vi "Main VI.vi"   [LabVIEW 2017]
uses:
  Main Flow.ctl
types:
  T1 = typedef "Main Flow.ctl" = enum16{"Initialize", "Calibrate Max Threshold", "Wait for Signal", "Convert Signal", "Noise Processing", "Threshold Processing", "Stop"}
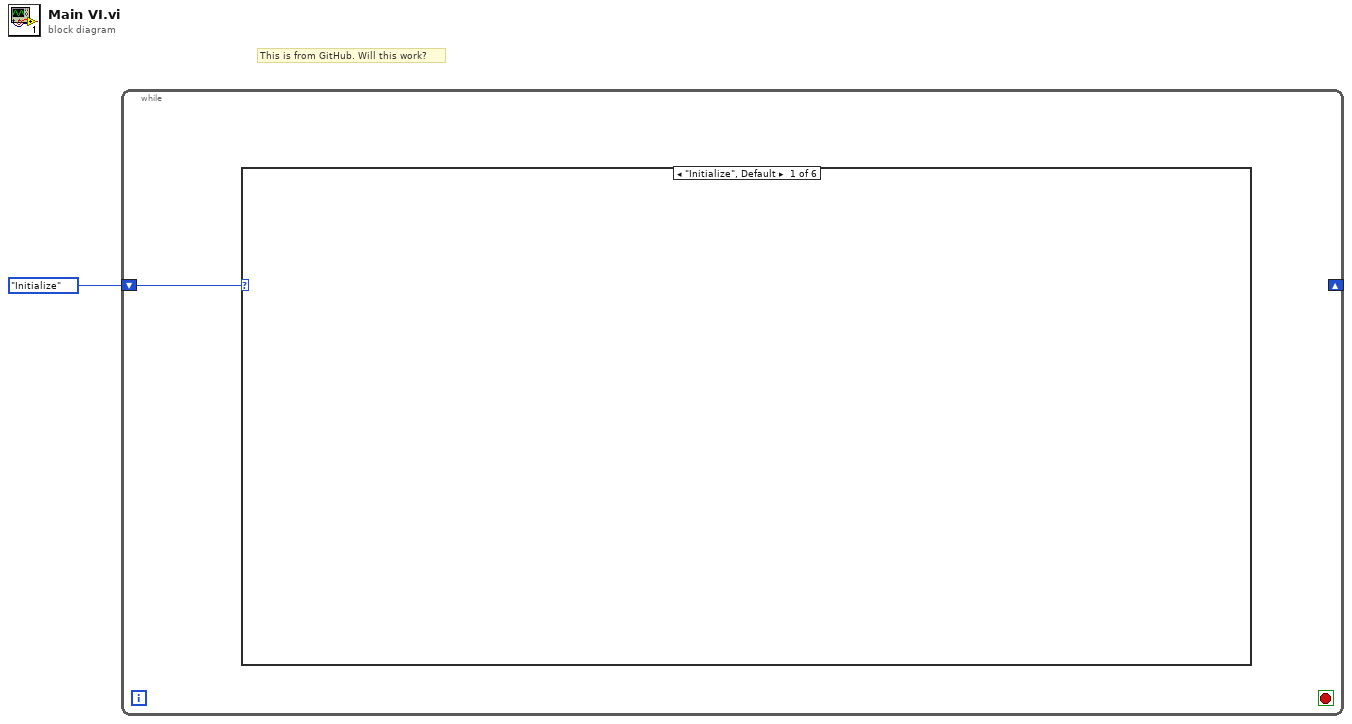
[diagram p0: block diagram]
diagram:
  # "This is from GitHub. Will this work?"
  n1 = while {
    shift-right: _ -> [_]
    shift-left: Main_Flow."Initialize" -> [w2]
    stop <- _ stop-if-true
    n2 = case shown="\"Initialize\", Default" w2 {
      frame "Initialize", Default {
      }
      frame "Calibrate Max Threshold" {
      }
      frame "Wait for Signal" {
      }
      frame "Noise Processing" {
      }
      frame "Threshold Processing" {
      }
      frame "Stop" {
      }
    }
  }
